vi "Grad_a_Rad.vi"(1 "Grados":dbl) -> (0 "Radianes":dbl)   [LabVIEW 2020]
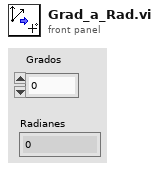
[diagram p1: front panel]
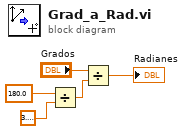
[diagram p0: block diagram]
diagram:
  n1 = Divide(x=180.0 ("y"), y=3.141592653589793) -> (x/y=w4:dbl)
  n2 = Divide(x="Grados", y=w4) -> (x/y=→"Radianes":dbl)
